vi "Remove Separator and Whitspace.vi"(11 "Table string":string) -> (3 "Trimmed string":string)   [LabVIEW 2021]
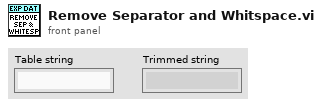
[diagram p1: front panel]
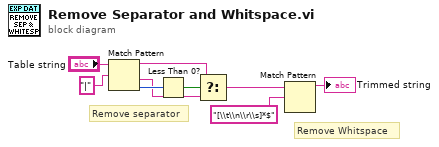
[diagram p0: block diagram]
diagram:
  # "Remove Whitspace"
  # "Remove separator"
  n1 = Match Pattern(string="Table string", regular expression="|") -> (before substring=w1:string, after substring=w6:string, offset past match=w8:i32)  [unwired: 1 in, 1 out]
  n2 = Less Than 0?(x=w8) -> (x < 0?=w7:bool)
  n3 = Select(t=w1, s=w7, f=w6) -> (s? t:f=w5:string)
  n4 = Match Pattern(string=w5, regular expression="[\\t\\n\\r\\s]*$") -> (before substring=→"Trimmed string":string)  [unwired: 1 in, 3 out]
